vi "Auto-Write to Folder and file for Blank_YCC.vi"(5 "Who's Data":enum16{"YCC", "PYW", "LCH", "YYH"}(ring), 6 "data to be saved":dbl[][](array[numeric]) format="%0.2f", 7 "File name add to the end \n(height)":string="h300", 8 "Title":string="-UnfoldedOnly-", 9 "Save?":bool) -> (2 "Save to File Name":string, 3 "Save to Path":path)   [LabVIEW 2014]
uses:
  Main-Stage-Based/(Global) Current handle and LaserPower_YCC.vi
  <vilib>/Utility/file.llb/Write To Spreadsheet File (DBL).vi
panel:
  out "Folder name":string
  out "folder exists?":bool
  out "date/time string":string
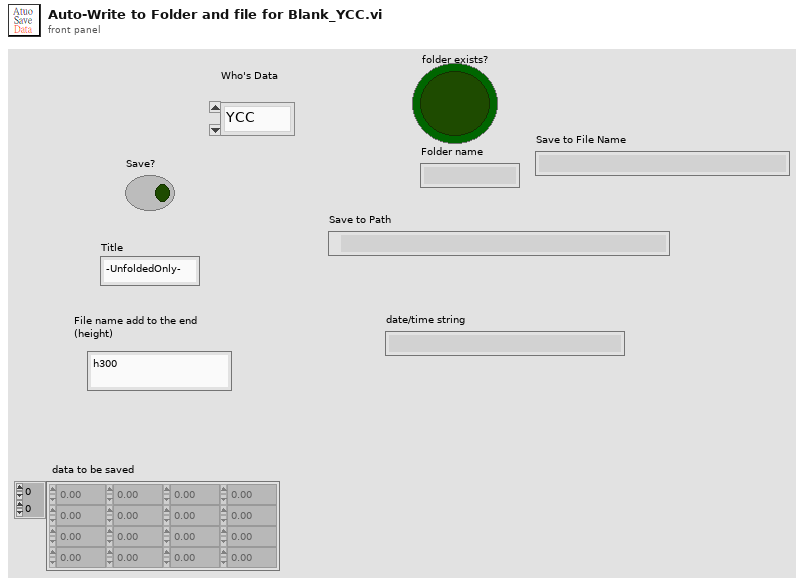
[diagram p1: front panel]
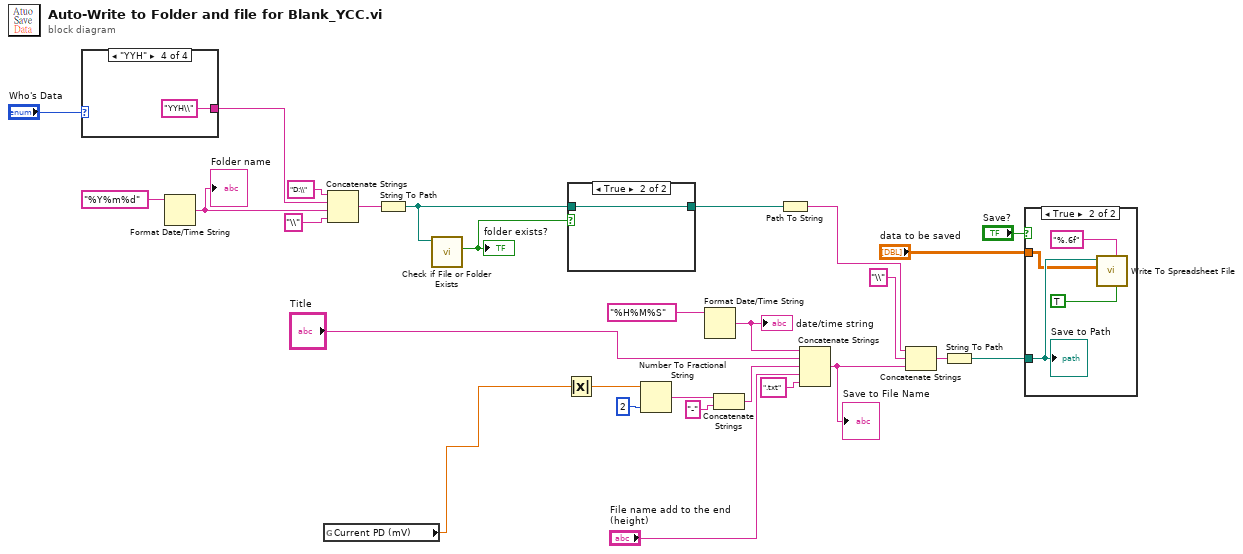
[diagram p0: block diagram]
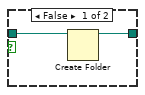
[diagram p2: hidden frame]
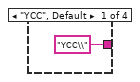
[diagram p4: hidden frame]
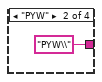
[diagram p5: hidden frame]
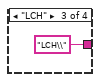
[diagram p6: hidden frame]
diagram:
  n1 = case shown="\"YYH\"" "Who's Data" {
    tunnel: ["YCC\\" ("string") "PYW\\" ("string") "LCH\\" ("string") "YYH\\" ("string")] -> w26
    frame "YCC", Default {
    }
    frame "PYW" {
    }
    frame "LCH" {
    }
    frame "YYH" {
    }
  }
  n2 = Format Date/Time String(time format string (%c)="%Y%m%d") -> (date/time string=w13:string)  [unwired: 2 in]
  "Folder name" <- w13
  n3 = global read "(Global) Current handle and LaserPower_YCC.vi" "Current PD (mV)"() -> (w1:dbl)
  n4 = Concatenate Strings("D:\\" ("string"), w26, w13, "\\" ("string")) -> (w25:string)
  n5 = String To Path(string=w25) -> (path=w16:path)
  n6 = call <vilib>:"Check if File or Folder Exists.vi"("path"=w16) -> ("file or folder exists?"=w15:bool)  [unwired: 8 in, 2 out]
  "folder exists?" <- w15
  n7 = Absolute Value(x=w1) -> (abs(x)=w2:dbl)
  n8 = case shown="True" w15 {
    tunnel: w16 -> [w34 w35]
    tunnel: [w33 w35] -> w21
    frame False {
      n9 = Create Folder(path (use dialog)=w34) -> (created path=w33:path)  [unwired: 2 in, 2 out]
    }
    frame True {
    }
  }
  n10 = Number To Fractional String(number=w2, precision (6)=i16 2) -> (F-format string=w6:string)  [unwired: 2 in]
  n11 = Format Date/Time String(time format string (%c)="%H%M%S") -> (date/time string=w10:string)  [unwired: 2 in]
  "date/time string" <- w10
  n12 = Concatenate Strings(w6, "-" ("string")) -> (w4:string)
  n13 = Path To String(path=w21) -> (string=w18:string)
  n14 = Concatenate Strings(w10, "Title", w4, "File name add to the end \n(height)", ".txt" ("string")) -> (w12:string)
  "Save to File Name" <- w12
  n15 = Concatenate Strings(w18, "\\" ("string"), w12) -> (w20:string)
  n16 = String To Path(string=w20) -> (path=w19:path)
  n17 = case shown="True" "Save?" {
    tunnel: w19 -> [_ w38]
    tunnel: "data to be saved" -> [_ w37]
    frame False {
    }
    frame True {
      n18 = call-poly <vilib>:"Write To Spreadsheet File.vi"("transpose? (no:F)"=TRUE, "format (%.3f)"="%.6f", "2D data"=w37, "file path (dialog if empty)"=w38) -> ()  [unwired: 4 in, 1 out]
      "Save to Path" <- w38
    }
  }
